vi "analizzatore di spettro.vero.vi"() -> ()   [LabVIEW 2018]
uses:
  <vilib>/Analysis/4window.llb/windowTd.ctl
  <vilib>/Utility/error.llb/DialogType.ctl
  <vilib>/measure/maspectr.llb/FFT Spectrum (Mag-Phase) for 1 Chan.vi
  <vilib>/measure/NI_MAPro.lvlib
  <vilib>/Analysis/NI_AALPro.lvlib
panel:
  in  "?":enum32{"start/stop", "centro & span"}(tab)
  in  "f start [Hz]":dbl min=0.0 step=1.0
  in  "f stop [Hz]":dbl=1000.0 min=0.0 step=1.0
  in  "Center freq":dbl=50.0 min=0.0 step=1.0 format="%0.2p"
  in  "span [Hz]":dbl=1.0 min=0.0 step=1.0 format="%0.2p"
  in  "df [Hz]":dbl=0.1
  out "fc [Hz]":dbl=51.2
  out "N":dbl=512.0
  in  "window":T1 items=["Rectangle"=0, "Hanning"=1, "Hamming"=2, "Blackman-Harris"=3, "Exact Blackman"=4, "Blackman"=5, "Flat Top"=6, "4 Term B-Harris "=7, "7 Term B-Harris"=8, "Low Sidelobe"=9, "Blackman Nuttall"=11, "Triangle"=30, "Bartlett-Hanning"=31, "Bohman"=32, "Parzen"=33, "Welch"=34, "Kaiser"=60, "Dolph-Chebyshev"=61, "Gaussian"=62]
  in  "scala y":string(combo)="linear"
  in  "frequency":string(combo)="start/stop"
  in  "stop":bool
  out "spettro di frequenza":cluster{"f0":dbl, "df":dbl, "magnitude":dbl[]}(graph)={"f0"=0.0, "df"=0.1, "magnitude"=[0.016212089775900506, 3.462161787985884e-05, 1.7423020864752125e-05, 1.9003433680266948e-05, 1.6825271207022547e-05, 3.580379439861196e-05, 1.824317393040275e-05, 4.511495932963334e-05, 5.388663877775837e-05, 4.7423255880640024e-05, 0.00018324483807227818, 1.4144322074317983, 0.00019422557921538853, 3.5862910945552426e-05, 8.087498937834196e-05, 8.05407025685909e-05, 6.734473785632877e-05, 4.21265493029532e-05, 6.600109619444197e-05, 4.426932402832496e-05, 4.838686365725399e-05, 1.699184147226685e-05, 0.00013903672094247384, 4.471042915314811e-05, 2.8669833956826474e-05, 4.5958034555521214e-05, 5.088077917555049e-05, 2.2156989087856475e-05, 2.6324324890319082e-05, 1.8715104134700513e-05, 2.1444085244662928e-05, 1.3729237241049758e-05, 2.612420434773621e-05, 3.226483671836953e-05, 3.901697525002169e-05, 4.0099711283498155e-05, 2.6663409711823823e-05, 3.538243471136227e-05, 5.484936541635876e-05, 2.6518603527349857e-05, 2.6457840628490816e-05, 1.4323931506934138e-05, 3.0583547842047614e-05, 2.0602624243470368e-05, 6.214170475727027e-05, 1.5272889690201525e-05, 4.45458299261378e-06, 1.8492608982150432e-05, 3.0538816723958872e-06, 1.3416567907234277e-05, 4.1949550129538245e-05, 2.2201702084702648e-05, 2.5069877643390437e-05, 3.452521031410338e-05, 6.395256469080979e-06, 3.293638013788603e-05, 2.4627157608956507e-06, 3.7310432257514945e-05, 9.818109743215654e-06, 2.399424316796938e-05, 1.3973060620180733e-06, 2.209906308846045e-05, 2.0065943073248314e-05, 2.175316226485824e-05, 3.526474001682725e-05, 1.5176854965220282e-05, 2.841287861080178e-05, 3.4480591977178806e-05, 1.3743315911194367e-05, 1.4025671164534152e-05, 2.27156172762778e-05, 1.4764572283262869e-05, 2.485694136259805e-05, 3.1531237127833774e-05, 1.8178349594436283e-05, 3.2029563694965306e-05, 5.7380475475656775e-05, 3.302495071208353e-05, 1.7295489885864845e-05, 2.1952947552736815e-05, 3.31083673313554e-05, 2.356200187375309e-05, 7.486244750115287e-06, 2.947383007674689e-05, 7.846660766062121e-06, 1.478496108509012e-05, 4.8268073407045876e-05, 7.670539182655471e-06, 1.97357208993591e-05, 2.1115240419642318e-05, 7.529322926078663e-06, 1.9626457829796482e-05, 6.986149046976143e-06, 2.6061810650564766e-05, 2.7368795641811363e-05, 2.5445669234853052e-05, 2.3055994489891257e-05, 1.4934938681780858e-05, 3.097492299548742e-05, 2.035038229470488e-05, 6.312392662954568e-06, 1.4328522261307315e-05, 2.3316779398195063e-05, 2.3097551245111524e-05, 3.210659722741828e-05, 1.253500408540657e-05, 2.1152337013003072e-05, 5.277380025362799e-06, 1.6932661927332502e-05, 1.5302349533510652e-05, 4.224246560449051e-05, 1.8286776691077583e-05, 2.4161313563557916e-05, 4.1504057069250605e-05, 2.205852953099762e-05, 1.6730951602752527e-05, 1.0633059839698966e-05, 1.2985650583629058e-05, 5.1227848673920754e-05, 7.154446720822012e-06, 5.647504555725167e-05, 4.5067415312517694e-05, 1.5114601712102046e-05, 1.243351207495508e-05, 3.7684994141509674e-05, 2.82227388420202e-06, 1.9393517618986314e-05, 3.4030615573456735e-05, 1.124188574864729e-05, 1.596419413105693e-05, 3.080118705173089e-05, 4.3488144464589326e-05, 7.363309045673461e-06, 1.875035019158976e-05, 4.039189164299144e-05, 4.467983772594492e-05, 8.185693699381152e-06, 1.3022621754319449e-05, 1.5708940145295882e-05, 1.1358818394774414e-05, 7.092163583198665e-06, 2.71190439097789e-05, 1.3906069350931973e-05, 2.948542704564951e-05, 1.8774849564648266e-05, 2.7341443040332127e-05, 4.551244515829423e-06, 1.3487437282933253e-05, 2.8658823349915857e-05, 1.1443685121647808e-05, 1.6244298820572316e-05, 6.564745469233553e-06, 3.274664431684394e-05, 1.76023237610363e-05, 1.1088519508348788e-05, 4.408320090433645e-05, 2.137871304392614e-05, 8.649323016297927e-06, 2.7163044751558925e-05, 4.884387130902338e-05, 7.25247609468276e-06, 2.3925186680258812e-05, 3.515902503387745e-05, 2.2286879462876476e-05, 1.0037163230259381e-05, 1.2572039850326964e-05, 5.171962260843198e-06, 6.622620908473186e-06, 1.332382120127983e-06, 4.1957505497952373e-05, 3.0038860256117344e-05, 2.6732653161530678e-05, 1.8780471060970192e-05, 1.185689478376351e-05, 2.8376285395133928e-05, 2.5439976096705482e-05, 2.965808697116915e-05, 4.7536661068570104e-05, 2.3369927310907182e-05, 2.735136438059478e-05, 3.237047207268064e-05, 1.7507098960017122e-05, 2.2270307755752918e-05, 4.275695905892627e-05, 2.0942340254831997e-05, 9.249639105823884e-06, 6.901400134043114e-06, 1.0764260660554263e-05, 2.274522478773075e-05, 6.428859097141312e-06, 3.486730243188847e-05, 1.3361644384829653e-05, 2.2270610504679168e-05, 2.281014557819611e-05, 1.6266959917315472e-05, 2.483911329310082e-05, 3.845625624862157e-06, 8.42508947434116e-06, 1.9403864227668376e-05, 5.751056797731486e-06, 2.619705505587515e-05, 4.749895204505905e-06, 2.904208764273048e-05, 2.4314472217774433e-05, 1.29970177078378e-05, 1.2439983769536339e-05, 5.65118581449865e-06, 8.72842136584306e-06, 1.2413896947999563e-06, 2.395963843260268e-05, 4.593844978091179e-06, 3.501587505884961e-05, 1.7093702061628902e-05, 1.98814463056302e-05, 2.256826119452526e-05, 2.2464530257004037e-05, 4.8062175856697065e-05, 2.800007741080796e-05, 7.815550749866445e-06, 2.4517925558097303e-05, 1.8744553283764303e-05, 4.921690047653588e-06, 1.9073396390056157e-05, 1.693088178532694e-05, 2.7424869536188926e-05, 2.4690610142194996e-05, 2.5893060829452902e-05, 2.1865988274283377e-05, 2.2482562476803645e-05, 3.658303704311097e-05, 1.1252387685416639e-05, 6.572042949221018e-06, 2.531474960895049e-05, 3.355878955631464e-05, 1.556444365885701e-05, 7.640941991427869e-06, 2.5824138087331726e-05, 3.867666684451173e-05, 9.060508254362069e-06, 2.2829523412372998e-05, 2.02984546144728e-05, 3.7959492194133805e-05, 3.3595220686419286e-05, 3.971158835776062e-05, 2.0762429856027843e-05, 2.6958053225253803e-05, 2.4333188177173732e-05, 4.546401577381655e-06, 2.1007780119112274e-05, 2.2236950285272962e-05, 3.8352499582069406e-05, 4.336223897005926e-05, 3.2754748164257e-05, 2.1745699427807856e-05, 1.764380913723096e-05, 1.5943614639346726e-05]}
  # "SPETTRO DI FREQUENZA"
  # "SPETTRO DI FREQUENZA"
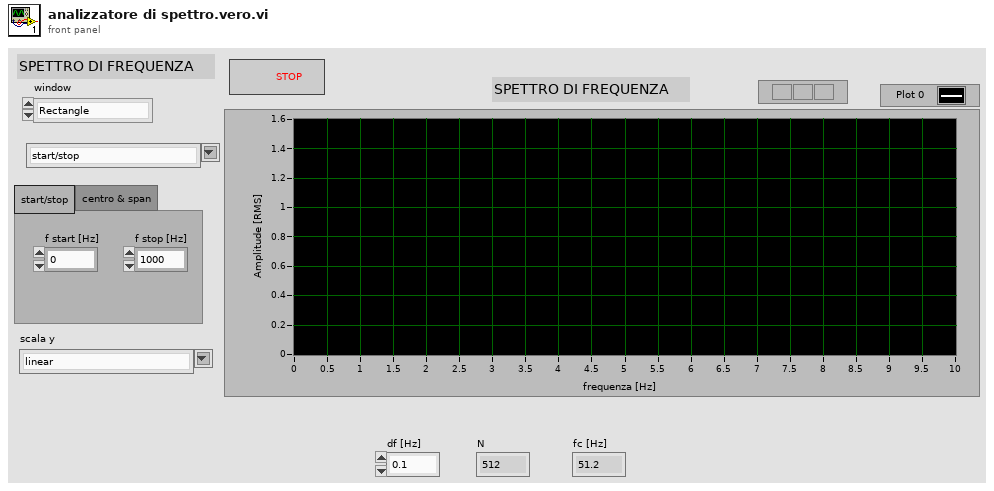
[diagram p1: front panel]
types:
  T1 = typedef "NI_AALPro.lvlib/windowTd.ctl" = u32
  T2 = typedef "DialogType.ctl" = u16
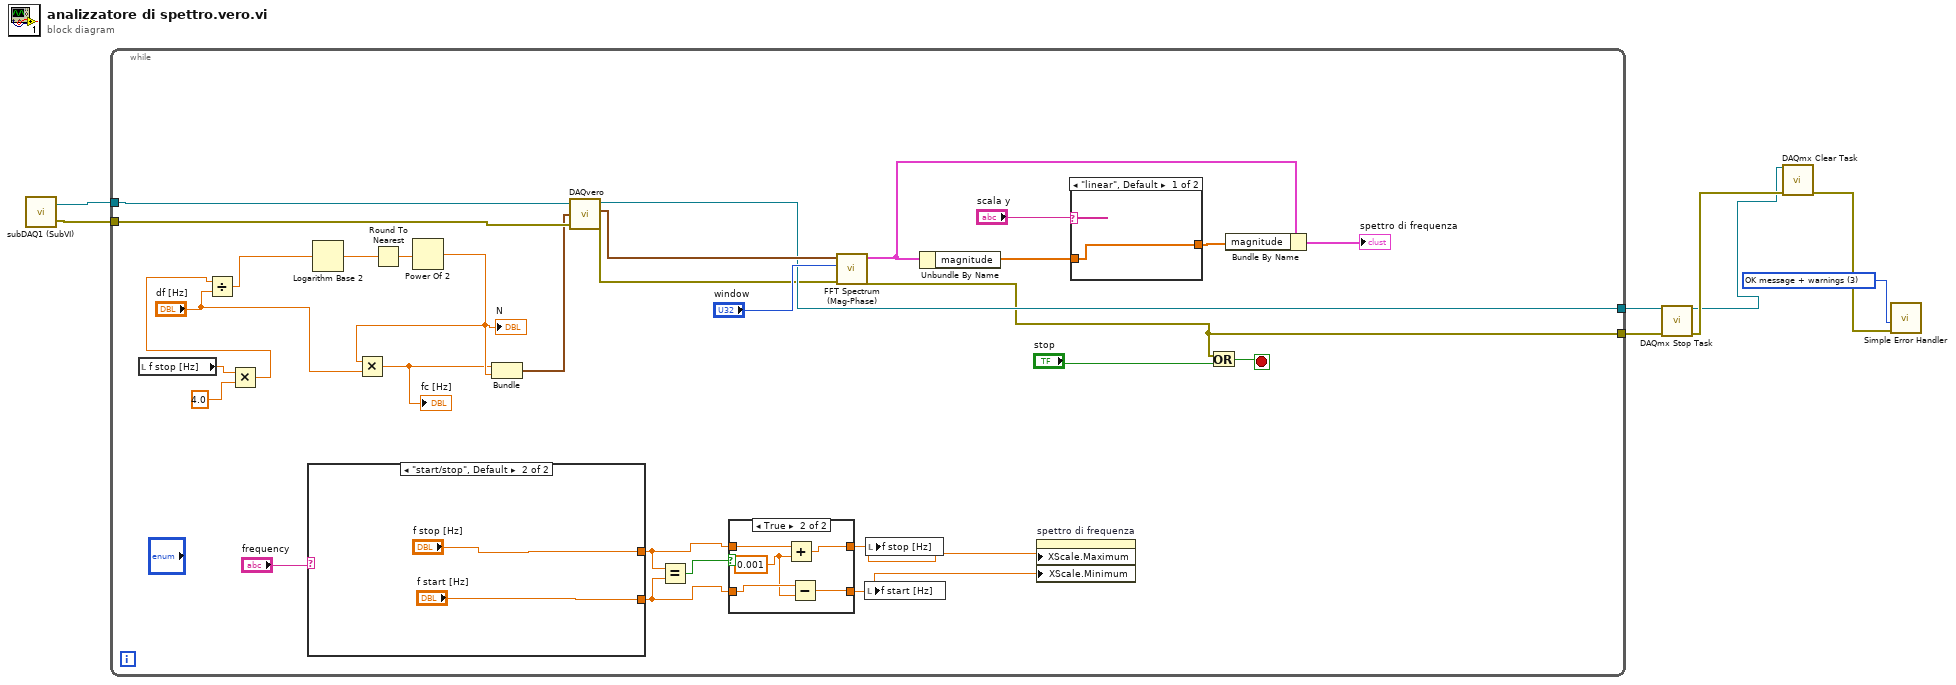
[diagram p0: block diagram]
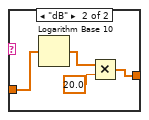
[diagram p3: hidden frame]
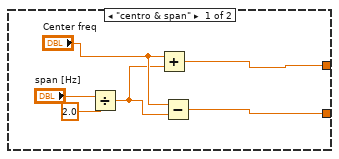
[diagram p4: hidden frame]
diagram:
  w3 = T2 3 items=["no dialog", "OK message", "continue or stop message", "OK message + warnings", "continue/stop + warnings"] ("type of dialog (OK msg:1)")
  n1 = call "subDAQ1 (SubVI).vi"() -> ("error out"=w7:errorcluster, "Refnum out"=w8:refnum<k21>)  [unwired: 3 in]
  n2 = while {
    tunnel: w8 -> [w24]
    tunnel: w7 -> [w23]
    tunnel: [w21] -> w2
    tunnel: [w19] -> w1
    stop <- w37 stop-if-true
    n3 = local read "f stop [Hz]"() -> (w13:dbl)
    n4 = Multiply(x=w13, y=4.0) -> (x*y=w14:dbl)
    n5 = Divide(x=w14, y="df [Hz]") -> (x/y=w18:dbl)
    n6 = case shown="\"start/stop\", Default" "frequency" {
      tunnel: [w52 "f stop [Hz]"] -> w32
      tunnel: [w51 "f start [Hz]"] -> w33
      frame "centro & span" {
        n7 = Divide(x="span [Hz]", y=2.0) -> (x/y=w53:dbl)
        n8 = Add(x="Center freq", y=w53) -> (x+y=w52:dbl)
        n9 = Subtract(x="Center freq", y=w53) -> (x-y=w51:dbl)
      }
      frame "start/stop", Default {
      }
    }
    n10 = Logarithm Base 2(1:w18) -> (0:w16:dbl)
    n11 = Round To Nearest(number=w16) -> (nearest integer value=w15:dbl)
    n12 = Power Of 2(x=w15) -> (2^x=w10:dbl)
    "N" <- w10
    n13 = Multiply(x=w10, y="df [Hz]") -> (x*y=w9:dbl)
    "fc [Hz]" <- w9
    n14 = Bundle(w9, w10) -> (w11:cluster{dbl, dbl})  [unwired: 1 in]
    n15 = call "DAQvero.vi"("task/channels in"=w24, "sampling info"=w11, "error in"=w23) -> ("task out"=w21:refnum<k21>, "1 segnale"=w22:waveform(dbl), "error out"=w20:errorcluster)  [unwired: 1 out]
    n16 = Equal?(x=w32, y=w33) -> (x = y?=w34:bool)
    n17 = case shown="True" w34 {
      tunnel: w33 -> [w39 w44]
      tunnel: w32 -> [w40 w45]
      tunnel: [w40 w41] -> w26
      tunnel: [w39 w42] -> w25
      frame False {
      }
      frame True {
        w43 = 0.001 ("y")
        n18 = Add(x=w45, y=w43) -> (x+y=w41:dbl)
        n19 = Subtract(x=w44, y=w43) -> (x-y=w42:dbl)
      }
    }
    n20 = call-poly <vilib>:"FFT Spectrum (Mag-Phase).vi"("error in (no error)"=w20, "window"="window", "time signal"=w22) -> ("error out"=w19:errorcluster, "magnitude"=w30:cluster{"f0":dbl, "df":dbl, "magnitude":dbl[]})  [unwired: 4 in, 3 out]
    n21 = local write "f start [Hz]"(w25) -> ()
    n22 = local write "f stop [Hz]"(w26) -> ()
    n23 = Unbundle By Name(w30) -> ("magnitude"=w29:dbl[])
    n24 = property on="spettro di frequenza" class="WFGraph (strict)"("XScale.Maximum"=w26, "XScale.Minimum"=w25) -> ()  [unwired: 2 in, 2 out]
    n25 = case shown="\"linear\", Default" "scala y" {
      tunnel: [w46 w48] -> w28
      tunnel: w29 -> [w46 w47]
      frame "linear", Default {
      }
      frame "dB" {
        n26 = Logarithm Base 10(1:w47) -> (0:w50:dbl[])
        n27 = Multiply(x=w50, y=20.0) -> (x*y=w48:dbl[])
      }
    }
    n28 = Or(x=w19, y="stop") -> (x .or. y?=w37:bool)
    n29 = Bundle By Name(cluster=w30, "magnitude"=w28) -> (→"spettro di frequenza":cluster{"f0":dbl, "df":dbl, "magnitude":dbl[]})
  }
  n30 = call <vilib>:"DAQmx Stop Task.vi"("task/channels in"=w2, "error in"=w1) -> ("task out"=w4:refnum<k21>, "error out"=w5:errorcluster)  [unwired: 12 in]
  n31 = call <vilib>:"DAQmx Clear Task.vi"("task in"=w4, "error in"=w5) -> ("error out"=w6:errorcluster)  [unwired: 13 in]
  n32 = call <vilib>:"Simple Error Handler.vi"("type of dialog (OK msg:1)"=w3, "error in (no error)"=w6) -> ()  [unwired: 3 in, 5 out]
